vi "Sertifika_Verilerini_Al.vi"() -> (0 "error out":errorcluster, 1 "Kalibrasyon Tarihi":string, 2 "GKC_Uretici":string, 3 "GKC_Tip":string, 4 "GKC_Seri_No":string, 5 "Cihazin_Sahibi":string, 6 "Ref_Seri_No":string, 7 "Kalibrasyonu_Yapan":string)   [LabVIEW 2014]
panel:
  in  "Enum":T1=enum."PQ++"
  in  "üretici":T2
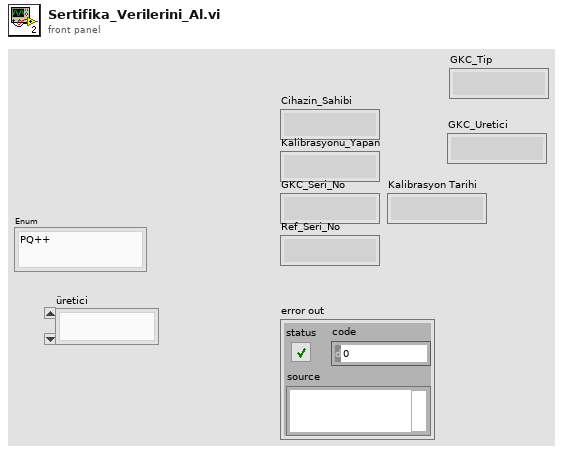
[diagram p1: front panel]
types:
  T1 = typedef "GKÇ_Tip.ctl" = enum16{"", "PQ+", "PQ++", "ION"}
  T2 = typedef "GKÇ_Uretici.ctl" = enum16{"", "TÜBİTAK EE", "SCHNEIDER"}
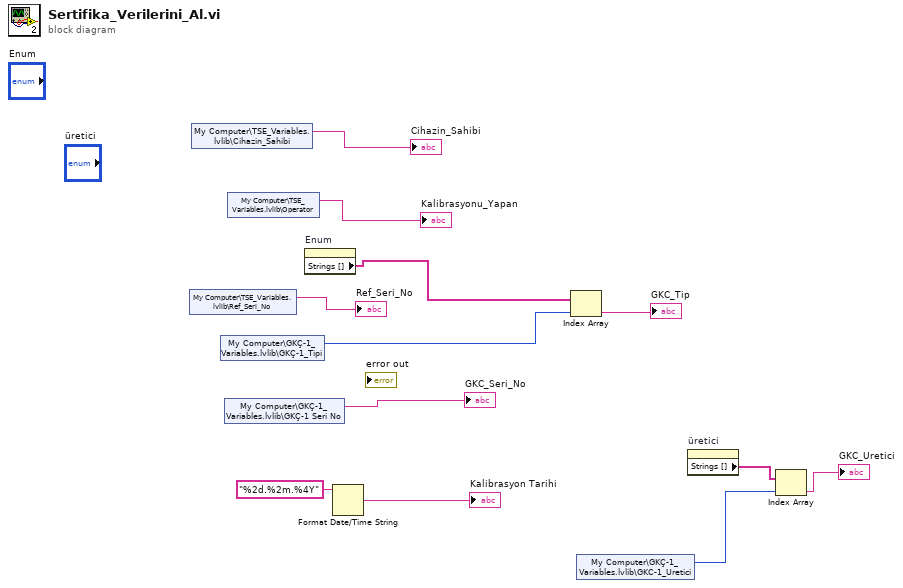
[diagram p0: block diagram]
diagram:
  n1 = shared-variable "My Computer\\TSE_Variables.lvlib\\Ref_Seri_No"() -> (→"Ref_Seri_No":string)  [unwired: 1 in, 1 out]
  n2 = shared-variable "My Computer\\TSE_Variables.lvlib\\Cihazin_Sahibi"() -> (→"Cihazin_Sahibi":string)  [unwired: 1 in, 1 out]
  n3 = shared-variable "My Computer\\GKÇ-1_Variables.lvlib\\GKÇ-1_Tipi"() -> (w6:T1)  [unwired: 1 in, 1 out]
  n4 = shared-variable "My Computer\\GKÇ-1_Variables.lvlib\\GKÇ-1 Seri No"() -> (→"GKC_Seri_No":string)  [unwired: 1 in, 1 out]
  n5 = shared-variable "My Computer\\TSE_Variables.lvlib\\Operator"() -> (→"Kalibrasyonu_Yapan":string)  [unwired: 1 in, 1 out]
  n6 = property on="Enum" class="Enum (strict)"() -> ("Strings []"=w1:string[])  [unwired: 2 in, 2 out]
  n7 = Format Date/Time String(time format string (%c)="%2d.%2m.%4Y") -> (date/time string=→"Kalibrasyon Tarihi":string)  [unwired: 2 in]
  n8 = Index Array(array=w1, index=w6) -> (element=→"GKC_Tip":string)
  n9 = shared-variable "My Computer\\GKÇ-1_Variables.lvlib\\GKC-1_Uretici"() -> (w3:T2)  [unwired: 1 in, 1 out]
  n10 = property on="üretici" class="Enum (strict)"() -> ("Strings []"=w4:string[])  [unwired: 2 in, 2 out]
  n11 = Index Array(array=w4, index=w3) -> (element=→"GKC_Uretici":string)
